vi "Teleop.vi"(10 "Match Info":T1={"Autonomous Elapsed Seconds"=0.0, "TeleOp Elapsed Seconds"=0.0, "Disabled Elapsed Seconds"=0.0, "Visited Autonomous"=FALSE, "Visited TeleOp"=FALSE, "Visited Disabled"=FALSE, "Autonomous Settings"={"Autonomous Style"=enum."Independent", "VI Refnum"=refnum}}, 11 "Call Context":T2) -> ()   [LabVIEW 2014]
doc: "This VI is called for each TeleOp packet received from the DS where the robot is not disabled. It is often used to read from the joysticks and update I/O or to update setpoints for timed control loops. It should complete and return within 20 milliseconds or it may miss DS packets."
uses:
  <vilib>/Rock Robotics/WPI/DriverStation/WPI_DriverStationDerivedRobotMode.ctl
  <vilib>/Rock Robotics/WPI/DriverStation/WPI_DriverStationMatch Info.ctl
  <vilib>/Rock Robotics/Network Tables/SD Read Boolean.vi
  <vilib>/Rock Robotics/Network Tables/SD Read Number.vi
  <vilib>/Rock Robotics/WPI/RobotDrive/WPI_RobotDriveGetSetRefNum.vi
  <vilib>/Rock Robotics/WPI/Joystick/WPI_JoystickGetSetRefNum.vi
  <vilib>/Rock Robotics/Network Tables/SD Write Boolean Array.vi
  <vilib>/Rock Robotics/Network Tables/SD Write Numeric Array.vi
  <vilib>/Rock Robotics/WPI/RobotDrive/WPI_RobotDriveArcadeDrive_Standard(NoSaturation).vi
  Robot Global Data.vi
  <vilib>/Rock Robotics/WPI/Solenoid/WPI_SolenoidValue.ctl
  <vilib>/addons/control/pid/NI_PID_pid.lvlib
  <vilib>/Rock Robotics/WPI/Solenoid/WPI_SolenoidSetEnum.vi
  <vilib>/addons/control/pid/pid.llb/PID (DBL).vi
panel:
  out "EncoderDistance":dbl
  out "GyroAngle":dbl
  out "ArmVoltage":dbl
  out "Sample Slider 0":dbl(slide) scale=0.0..5.0
  out "Sample Boolean 1":bool
  out "Sample Boolean 0":bool
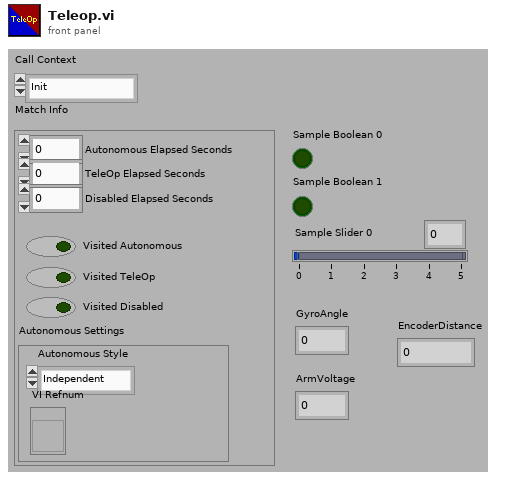
[diagram p1: front panel]
types:
  T1 = typedef "WPI_DriverStationMatch Info.ctl" = cluster{"Autonomous Elapsed Seconds":dbl, "TeleOp Elapsed Seconds":dbl, "Disabled Elapsed Seconds":dbl, "Visited Autonomous":bool, "Visited TeleOp":bool, "Visited Disabled":bool, "Autonomous Settings":cluster{"Autonomous Style":enum16{"Iterative", "Independent"}, "VI Refnum":refnum<vi>}}
  T2 = typedef "WPI_DriverStationDerivedRobotMode.ctl" = enum16{"Init", "Execute", "Stop"}
  T3 = typedef "WPI_JoystickDevRef.ctl" = cluster{"Device":T4}
  T4 = typedef "WPI_JoystickDeviceEnum.ctl" = enum16{"USB 0", "USB 1", "USB 2", "USB 3", "USB 4", "USB 5"}
  T5 = typedef "WPI_SolenoidValue.ctl" = enum16{"Off", "On", "Forward", "Reverse"}
  T6 = typedef "WPI_SolenoidDevRef.ctl" = cluster{"DevStatus":errorcluster, "Pneumatics Control Module":u8, "Forward Solenoid Channel":T7, "Reverse Solenoid Channel":T7}
  T7 = typedef "WPI_SolenoidChannel.ctl" = enum8{"Solenoid 0", "Solenoid 1", "Solenoid 2", "Solenoid 3", "Solenoid 4", "Solenoid 5", "Solenoid 6", "Solenoid 7", "Invalid"}
  T8 = cluster{"proportional gain (Kc)":dbl, "integral time (Ti, min)":dbl, "derivative time (Td, min)":dbl}
  T9 = typedef "WPI_AnalogChannelDevRef.ctl" = cluster{"DevStatus":errorcluster, "Controller":T10, "Analog Channel":T11}
  T10 = typedef "FPGA_TypedefAnalogModule.ctl" = enum16{"Controller 1"}
  T11 = typedef "FPGA_AIChannel.ctl" = enum8{"AI 0", "AI 1", "AI 2", "AI 3", "AI MXP 0", "AI MXP 1", "AI MXP 2", "AI MXP 3", "Invalid"}
  T12 = typedef "WPI_MotorControlDeviceRef.ctl" = cluster{"DeviceStatus":errorcluster, "Type":T13, "PWM":cluster{"Controller":T14, "PWM Channel":T15, "DeadBand":T16}, "CAN":cluster{"Device Number":u8, "Control Mode":T17, "Semaphore":T18, "Max Vout":dbl, "TalonSRX Control Mode":T19}, "Invert":bool, "TransformRef":T20, "InvTransformRef":T20}
  T13 = typedef "WPI_MotorControlType.ctl" = enum16{"PWM", "CAN", "CANTalonSRX"}
  T14 = typedef "FPGA_TypedefDigitalModule.ctl" = enum16{"Controller 1"}
  T15 = typedef "FPGA_DIOPWMChannel.ctl" = enum8{"PWM 0", "PWM 1", "PWM 2", "PWM 3", "PWM 4", "PWM 5", "PWM 6", "PWM 7", "PWM 8", "PWM 9", "PWM MXP 0", "PWM MXP 1", "PWM MXP 2", "PWM MXP 3", "PWM MXP 4", "PWM MXP 5", "PWM MXP 6", "PWM MXP 7", "PWM MXP 8", "PWM MXP 9", "Invalid"}
  T16 = typedef "WPI_PWMDeadband.ctl" = cluster{"Name":string, "maxPositivePwm":i32, "minPositivePwm":i32, "centerPwm":i32, "maxNegativePwm":i32, "minNegativePwm":i32, "angularRange":u16}
  T17 = typedef "WPI_CANJaguar_ControlMode.ctl" = enum8{"Percent VBus", "Current", "Speed", "Position", "Voltage"}
  T18 = typedef "Semaphore RefNum" = refnum<k1>
  T19 = typedef "WPI_CANTalonSRX_APIControlMode.ctl" = enum8{"Percent VBus", "Speed", "Position", "Slave", "Unchanged / Invalid"}
  T20 = typedef "WPI_PWMTransform_ConPane.ctl" = refnum<vi>
  T21 = typedef "WPI_RobotDriveDevRef.ctl" = cluster{"DevStatus":errorcluster, "Motors[]":T12[], "Square Inputs":bool, "Max Output":dbl}
  T22 = typedef "WPI_GyroDevRef.ctl" = cluster{"DevStatus":errorcluster, "Analog Module":T10, "Analog Channel":T11, "Offset":dbl, "Gain (VoltsPerDegree/Second)":dbl}
  T23 = typedef "WPI_EncoderDevRef.ctl" = cluster{"DevStatus":errorcluster, "EncoderIndex":T24, "CounterIndex":T25, "DistancePerCount":dbl, "Decoding Type":T26}
  T24 = typedef "FPGA_EncoderIdx.ctl" = enum8{"Enc 0", "Enc 1", "Enc 2", "Enc 3", "Enc 4", "Enc 5", "Enc 6", "Enc 7", "Invalid"}
  T25 = typedef "FPGA_CounterCtrSystemIndex.ctl" = enum8{"Ctr 0", "Ctr 1", "Ctr 2", "Ctr 3", "Ctr 4", "Ctr 5", "Ctr 6", "Ctr 7", "Invalid"}
  T26 = typedef "WPI_EncoderType.ctl" = enum16{"1x", "2x", "4x"}
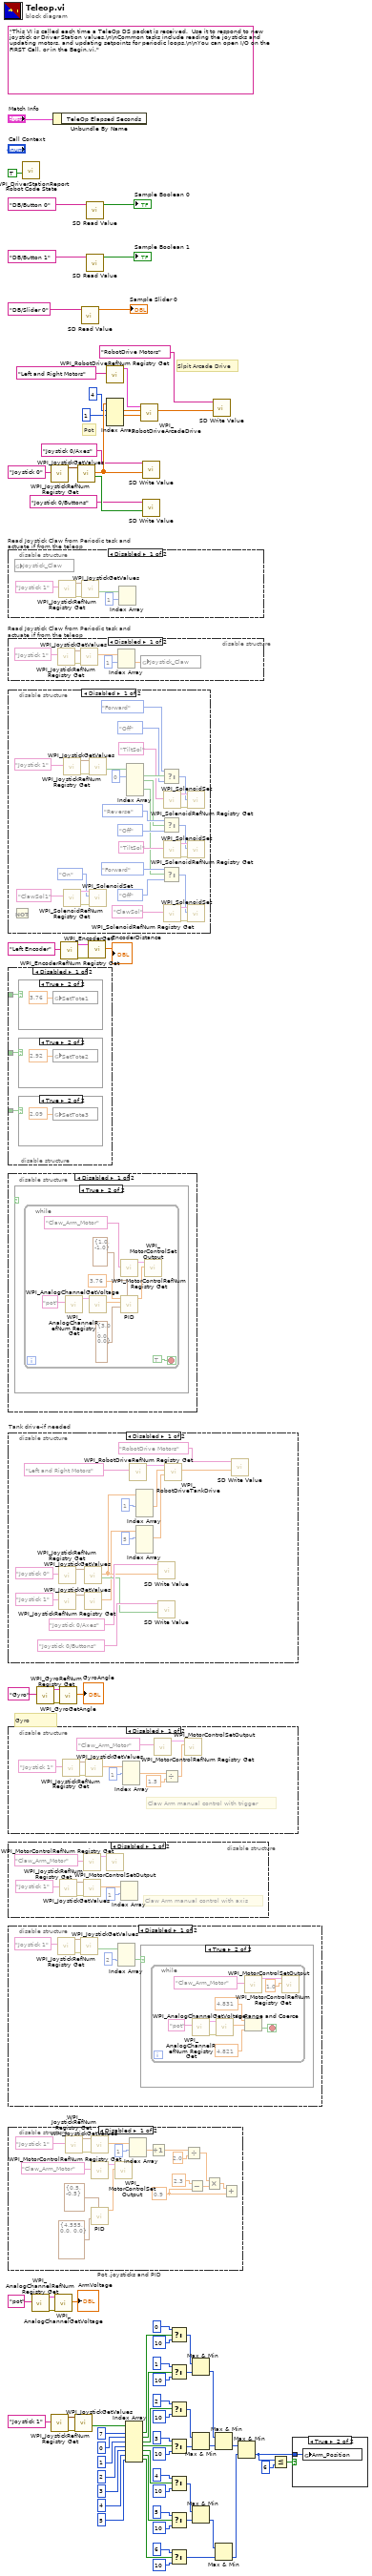
[diagram p0: block diagram]
diagram:
  (unwired) "This VI is called each time a TeleOp DS packet is received.  Use it to respond to new joystick or Driver Station values.\n\nCommon tasks include reading the joysticks and updating motors, and updating setpoints for periodic loops.\n\nYou can open I/O on the FIRST Call, or in the Begin.vi."
  # "Gyro"
  # "Pot"
  # "Slpit Arcade Drive"
  n1 = disable-structure "Read Joystick Claw from Periodic task and actuate if from the teleop" shown="Disabled" {
    frame Disabled {
      n2 = global read "Robot Global Data.vi" "Joystick_Claw"() -> ()  [unwired: 1 in]
      n3 = call <vilib>:"WPI_JoystickRefNum Registry Get.vi"("refnum name"="Joystick 1") -> ("error out"=w85:errorcluster, "JoystickDevRef"=w84:T3)  [unwired: 1 in, 8 out]
      n4 = call <vilib>:"WPI_JoystickGetValues.vi"("error in (no error)"=w85, "JoystickDevRef"=w84) -> ("Buttons"=w82:bool[])  [unwired: 5 in, 4 out]
      n5 = Index Array(array=w82, index #1=1 ("index")) -> ()  [unwired: 1 in, 2 out]
    }
    frame Enabled {
    }
  }
  n6 = disable-structure "Read Joystick Claw from Periodic task and actuate if from the teleop" shown="Disabled" {
    frame Disabled {
      n7 = call <vilib>:"WPI_JoystickRefNum Registry Get.vi"("refnum name"="Joystick 1") -> ("error out"=w90:errorcluster, "JoystickDevRef"=w89:T3)  [unwired: 1 in, 8 out]
      n8 = call <vilib>:"WPI_JoystickGetValues.vi"("error in (no error)"=w90, "JoystickDevRef"=w89) -> ("Axes"=w91:dbl[])  [unwired: 5 in, 4 out]
      n9 = Index Array(array=w91, index #1=1 ("index")) -> (element #1=w87:dbl)  [unwired: 1 in, 1 out]
      n10 = global write "Robot Global Data.vi" "Joystick_Claw"(w87) -> ()
    }
    frame Enabled {
    }
  }
  n11 = disable-structure shown="Disabled" {
    frame Disabled {
      n12 = Not() -> ()  [unwired: 1 in, 1 out]
      n13 = call <vilib>:"WPI_JoystickRefNum Registry Get.vi"("refnum name"="Joystick 1") -> ("error out"=w120:errorcluster, "JoystickDevRef"=w119:T3)  [unwired: 9 in]
      n14 = call <vilib>:"WPI_SolenoidRefNum Registry Get.vi"("refnum name"="ClawSol1") -> ("error out"=w101:errorcluster, "SolenoidDevRef"=w102:T6)  [unwired: 9 in]
      n15 = call <vilib>:"WPI_JoystickGetValues.vi"("error in (no error)"=w120, "JoystickDevRef"=w119) -> ("Buttons"=w112:bool[])  [unwired: 5 in, 4 out]
      n16 = call-poly <vilib>:"WPI_SolenoidSet.vi"("error in (no error)"=w101, "Value"=WPI_SolenoidValue."On", "SolenoidDevRef"=w102) -> ()  [unwired: 7 in, 2 out]
      n17 = Index Array(array=w112, index #1=0 ("index")) -> (element #1=w117:bool, element #2=w104:bool, element #4=w94:bool)  [unwired: 4 in, 2 out]
      n18 = Select(t=WPI_SolenoidValue."Forward", s=w117, f=WPI_SolenoidValue."Off" ("Value")) -> (s? t:f=w115:T5)
      n19 = Select(t=WPI_SolenoidValue."Reverse", s=w104, f=WPI_SolenoidValue."Off" ("Value")) -> (s? t:f=w107:T5)
      n20 = Select(t=WPI_SolenoidValue."Forward", s=w94, f=WPI_SolenoidValue."Off" ("Value")) -> (s? t:f=w97:T5)
      n21 = call <vilib>:"WPI_SolenoidRefNum Registry Get.vi"("refnum name"="TiltSol") -> ("error out"=w122:errorcluster, "SolenoidDevRef"=w121:T6)  [unwired: 9 in]
      n22 = call <vilib>:"WPI_SolenoidRefNum Registry Get.vi"("refnum name"="TiltSol") -> ("error out"=w108:errorcluster, "SolenoidDevRef"=w109:T6)  [unwired: 9 in]
      n23 = call <vilib>:"WPI_SolenoidRefNum Registry Get.vi"("refnum name"="ClawSol") -> ("error out"=w100:errorcluster, "SolenoidDevRef"=w99:T6)  [unwired: 9 in]
      n24 = call-poly <vilib>:"WPI_SolenoidSet.vi"("error in (no error)"=w122, "Value"=w115, "SolenoidDevRef"=w121) -> ()  [unwired: 7 in, 2 out]
      n25 = call-poly <vilib>:"WPI_SolenoidSet.vi"("error in (no error)"=w108, "Value"=w107, "SolenoidDevRef"=w109) -> ()  [unwired: 7 in, 2 out]
      n26 = call-poly <vilib>:"WPI_SolenoidSet.vi"("error in (no error)"=w100, "Value"=w97, "SolenoidDevRef"=w99) -> ()  [unwired: 7 in, 2 out]
    }
    frame Enabled {
    }
  }
  n27 = disable-structure shown="Disabled" {
    disable-tunnel: _ -> [w125 _]
    disable-tunnel: _ -> [w124 _]
    disable-tunnel: _ -> [w123 _]
    frame Disabled {
      n28 = case shown="True" w125 {
        frame False {
        }
        frame True {
          n29 = global write "Robot Global Data.vi" "SetTote1"(3.76 ("SetTote1")) -> ()
        }
      }
      n30 = case shown="True" w124 {
        frame False {
        }
        frame True {
          n31 = global write "Robot Global Data.vi" "SetTote2"(2.92 ("SetTote2")) -> ()
        }
      }
      n32 = case shown="True" w123 {
        frame False {
        }
        frame True {
          n33 = global write "Robot Global Data.vi" "SetTote3"(2.09 ("SetTote3")) -> ()
        }
      }
    }
    frame Enabled {
    }
  }
  n34 = disable-structure shown="Disabled" {
    frame Disabled {
      n35 = case shown="True" {
        selector: _ -> [_ _]
        frame False {
        }
        frame True {
          n36 = while {
            stop <- TRUE stop-if-true
            n37 = call <vilib>:"WPI_AnalogChannelRefNum Registry Get.vi"("refnum name"="pot") -> ("AIDeviceRef"=w132:T9)  [unwired: 9 in, 1 out]
            n38 = call <vilib>:"WPI_AnalogChannelGetVoltage.vi"("AIDeviceRef"=w132) -> ("Voltage"=w138:dbl)  [unwired: 1 in, 9 out]
            n39 = call <vilib>:"WPI_MotorControlRefNum Registry Get.vi"("refnum name"="Claw_Arm_Motor") -> ("MotorControlDevRef"=w135:T12)  [unwired: 1 in, 9 out]
            n40 = call-poly <vilib>:"PID.vi"("output range"=cluster{"output high":dbl, "output low":dbl} {"output high"=1.0, "output low"=-1.0}, "PID gains"=T8 {"proportional gain (Kc)"=3.0, "integral time (Ti, min)"=0.0, "derivative time (Td, min)"=0.0}, "process variable"=w138, "setpoint"=3.76 ("SetTote1")) -> ("output"=w130:dbl)  [unwired: 2 in, 5 out]
            n41 = call <vilib>:"WPI_MotorControlSetOutput.vi"("Output"=w130, "MotorControlDevRef"=w135) -> ()  [unwired: 2 in, 8 out]
          }
        }
      }
    }
    frame Enabled {
    }
  }
  n42 = disable-structure "Tank drive-if needed" shown="Disabled" {
    frame Disabled {
      n43 = call <vilib>:"WPI_JoystickRefNum Registry Get.vi"("refnum name"="Joystick 0") -> ("JoystickDevRef"=w153:T3)  [unwired: 1 in, 9 out]
      n44 = call <vilib>:"WPI_JoystickRefNum Registry Get.vi"("refnum name"="Joystick 1") -> ("JoystickDevRef"=w143:T3)  [unwired: 1 in, 9 out]
      n45 = call <vilib>:"WPI_JoystickGetValues.vi"("JoystickDevRef"=w143) -> ("Axes"=w144:dbl[])  [unwired: 6 in, 4 out]
      n46 = call <vilib>:"WPI_JoystickGetValues.vi"("JoystickDevRef"=w153) -> ("Buttons"=w148:bool[], "Axes"=w150:dbl[])  [unwired: 6 in, 3 out]
      n47 = call <vilib>:"WPI_RobotDriveRefNum Registry Get.vi"("refnum name"="Left and Right Motors") -> ("RobotDriveDevRef"=w147:T21)  [unwired: 1 in, 9 out]
      n48 = Index Array(array=w150, index #2=1 ("index")) -> (element #2=w145:dbl)  [unwired: 3 in, 3 out]
      n49 = Index Array(array=w144, index #1=5 ("index")) -> (element #1=w140:dbl)  [unwired: 3 in, 3 out]
      n50 = call-poly <vilib>:"SD Write Value.vi"("Numeric Array"=w150, "Name"="Joystick 0/Axes") -> ()  [unwired: 8 in, 2 out]
      n51 = call-poly <vilib>:"SD Write Value.vi"("Boolean Array"=w148, "Name"="Joystick 0/Buttons") -> ()  [unwired: 8 in, 2 out]
      n52 = call <vilib>:"WPI_RobotDriveTankDrive.vi"("Right axis value"=w140, "Left axis value"=w145, "RobotDriveDevRef"=w147) -> ("Motor Values"=w139:dbl[])  [unwired: 6 in, 2 out]
      n53 = call-poly <vilib>:"SD Write Value.vi"("Numeric Array"=w139, "Name"="RobotDrive Motors") -> ()  [unwired: 8 in, 2 out]
    }
    frame Enabled {
    }
  }
  n54 = disable-structure shown="Disabled" {
    frame Disabled {
      # "Claw Arm manual control with trigger"
      n55 = call <vilib>:"WPI_JoystickRefNum Registry Get.vi"("refnum name"="Joystick 1") -> ("error out"=w163:errorcluster, "JoystickDevRef"=w164:T3)  [unwired: 1 in, 8 out]
      n56 = call <vilib>:"WPI_JoystickGetValues.vi"("error in (no error)"=w163, "JoystickDevRef"=w164) -> ("Axes"=w160:dbl[])  [unwired: 5 in, 4 out]
      n57 = Index Array(array=w160, index #1=1 ("index")) -> (element #1=w158:dbl)  [unwired: 2 in, 2 out]
      n58 = call <vilib>:"WPI_MotorControlRefNum Registry Get.vi"("refnum name"="Claw_Arm_Motor") -> ("MotorControlDevRef"=w161:T12)  [unwired: 1 in, 9 out]
      n59 = Divide(x=w158, y=1.5) -> (x/y=w156:dbl)
      n60 = call <vilib>:"WPI_MotorControlSetOutput.vi"("Output"=w156, "MotorControlDevRef"=w161) -> ()  [unwired: 2 in, 8 out]
    }
    frame Enabled {
    }
  }
  n61 = disable-structure shown="Disabled" {
    frame Disabled {
      # "Claw Arm manual control with axis"
      n62 = call <vilib>:"WPI_JoystickRefNum Registry Get.vi"("refnum name"="Joystick 1") -> ("error out"=w168:errorcluster, "JoystickDevRef"=w167:T3)  [unwired: 1 in, 8 out]
      n63 = call <vilib>:"WPI_MotorControlRefNum Registry Get.vi"("refnum name"="Claw_Arm_Motor") -> ("MotorControlDevRef"=w170:T12)  [unwired: 1 in, 9 out]
      n64 = call <vilib>:"WPI_JoystickGetValues.vi"("error in (no error)"=w168, "JoystickDevRef"=w167) -> ("Axes"=w171:dbl[])  [unwired: 5 in, 4 out]
      n65 = call <vilib>:"WPI_MotorControlSetOutput.vi"("MotorControlDevRef"=w170) -> ()  [unwired: 3 in, 8 out]
      n66 = Index Array(array=w171, index #1=1 ("index")) -> ()  [unwired: 1 in, 2 out]
    }
    frame Enabled {
    }
  }
  n67 = disable-structure shown="Disabled" {
    frame Disabled {
      n68 = call <vilib>:"WPI_JoystickRefNum Registry Get.vi"("refnum name"="Joystick 1") -> ("error out"=w176:errorcluster, "JoystickDevRef"=w177:T3)  [unwired: 1 in, 8 out]
      n69 = call <vilib>:"WPI_JoystickGetValues.vi"("error in (no error)"=w176, "JoystickDevRef"=w177) -> ("Buttons"=w175:bool[])  [unwired: 5 in, 4 out]
      n70 = Index Array(array=w175, index #2=2 ("index")) -> (element #2=w174:bool)  [unwired: 2 in, 2 out]
      n71 = case shown="True" w174 {
        frame False {
        }
        frame True {
          n72 = while {
            stop <- w179 stop-if-true
            n73 = call <vilib>:"WPI_AnalogChannelRefNum Registry Get.vi"("refnum name"="pot") -> ("error out"=w185:errorcluster, "AIDeviceRef"=w184:T9)  [unwired: 9 in]
            n74 = call <vilib>:"WPI_AnalogChannelGetVoltage.vi"("error in (no error)"=w185, "AIDeviceRef"=w184) -> ("Voltage"=w180:dbl)  [unwired: 7 in, 2 out]
            n75 = call <vilib>:"WPI_MotorControlRefNum Registry Get.vi"("refnum name"="Claw_Arm_Motor") -> ("MotorControlDevRef"=w187:T12)  [unwired: 1 in, 9 out]
            n76 = In Range and Coerce(upper limit=4.831 ("lower limit"), x=w180, lower limit=4.821 ("upper limit")) -> (In Range?=w179:bool)  [unwired: 1 out]
            n77 = call <vilib>:"WPI_MotorControlSetOutput.vi"("Output"=1.0, "MotorControlDevRef"=w187) -> ()  [unwired: 2 in, 8 out]
          }
        }
      }
    }
    frame Enabled {
    }
  }
  n78 = disable-structure "Pot ,joysticks and PID" shown="Disabled" {
    frame Disabled {
      w194 = 0.9 ("y")
      n79 = call <vilib>:"WPI_JoystickRefNum Registry Get.vi"("refnum name"="Joystick 1") -> ("error out"=w204:errorcluster, "JoystickDevRef"=w203:T3)  [unwired: 1 in, 8 out]
      n80 = call <vilib>:"WPI_JoystickGetValues.vi"("error in (no error)"=w204, "JoystickDevRef"=w203) -> ("Axes"=w205:dbl[])  [unwired: 5 in, 4 out]
      n81 = call <vilib>:"WPI_MotorControlRefNum Registry Get.vi"("refnum name"="Claw_Arm_Motor") -> ("MotorControlDevRef"=w193:T12)  [unwired: 1 in, 9 out]
      n82 = call-poly <vilib>:"PID.vi"("output range"=cluster{"output high":dbl, "output low":dbl} {"output high"=0.5, "output low"=-0.5}, "PID gains"=T8 {"proportional gain (Kc)"=4.555, "integral time (Ti, min)"=0.0, "derivative time (Td, min)"=0.0}) -> ("output"=w189:dbl)  [unwired: 8 in, 1 out]
      n83 = call <vilib>:"WPI_MotorControlSetOutput.vi"("Output"=w189, "MotorControlDevRef"=w193) -> ()  [unwired: 2 in, 8 out]
      n84 = Index Array(array=w205, index #1=1 ("index")) -> (element #1=w201:dbl)  [unwired: 1 in, 1 out]
      n85 = Increment(x=w201) -> (x+1=w200:dbl)
      n86 = Divide(x=w200, y=2.0) -> (x/y=w198:dbl)
      n87 = Subtract(x=2.3, y=w194) -> (x-y=w197:dbl)
      n88 = Multiply(x=w198, y=w197) -> (x*y=w195:dbl)
      n89 = Add(x=w195, y=w194) -> ()  [unwired: 1 out]
    }
    frame Enabled {
    }
  }
  n90 = call <vilib>:"WPI_DriverStationReport Robot Code State.vi"("TeleOp"=TRUE ("Autonomous")) -> ()  [unwired: 10 in, 1 out]
  n91 = call <vilib>:"WPI_AnalogChannelRefNum Registry Get.vi"("refnum name"="pot") -> ("error out"=w54:errorcluster, "AIDeviceRef"=w55:T9)  [unwired: 9 in]
  n92 = call <vilib>:"WPI_GyroRefNum Registry Get.vi"("refnum name"="Gyro") -> ("error out"=w60:errorcluster, "GyroDevRef"=w59:T22)  [unwired: 9 in]
  n93 = call <vilib>:"WPI_JoystickRefNum Registry Get.vi"("refnum name"="Joystick 0") -> ("JoystickDevRef"=w67:T3)  [unwired: 1 in, 9 out]
  n94 = call <vilib>:"WPI_JoystickRefNum Registry Get.vi"("refnum name"="Joystick 1") -> ("error out"=w49:errorcluster, "JoystickDevRef"=w4:T3)  [unwired: 1 in, 8 out]
  n95 = Unbundle By Name("Match Info") -> ()  [unwired: 1 out]
  n96 = call <vilib>:"WPI_AnalogChannelGetVoltage.vi"("error in (no error)"=w54, "AIDeviceRef"=w55) -> ("Voltage"=→"ArmVoltage":dbl)  [unwired: 7 in, 2 out]
  n97 = call <vilib>:"WPI_GyroGetAngle.vi"("error in (no error)"=w60, "GyroDevRef"=w59) -> ("Angle"=→"GyroAngle":dbl)  [unwired: 6 in, 3 out]
  n98 = call <vilib>:"WPI_EncoderRefNum Registry Get.vi"("refnum name"="Left Encoder") -> ("error out"=w3:errorcluster, "EncoderDevRef"=w2:T23)  [unwired: 9 in]
  n99 = call <vilib>:"WPI_JoystickGetValues.vi"("error in (no error)"=w49, "JoystickDevRef"=w4) -> ("Buttons"=w47:bool[])  [unwired: 5 in, 4 out]
  n100 = call <vilib>:"WPI_JoystickGetValues.vi"("JoystickDevRef"=w67) -> ("Buttons"=w72:bool[], "Axes"=w70:dbl[])  [unwired: 6 in, 3 out]
  n101 = call-poly <vilib>:"SD Read Value.vi"("Name"="DB/Slider 0" ("refnum name")) -> ("Numeric"=→"Sample Slider 0":dbl)  [unwired: 8 in, 2 out]
  n102 = call-poly <vilib>:"SD Read Value.vi"("Name"="DB/Button 0" ("refnum name")) -> ("Boolean"=→"Sample Boolean 0":bool)  [unwired: 8 in, 2 out]
  n103 = call-poly <vilib>:"SD Read Value.vi"("Name"="DB/Button 1" ("refnum name")) -> ("Boolean"=→"Sample Boolean 1":bool)  [unwired: 8 in, 2 out]
  n104 = call <vilib>:"WPI_EncoderGet.vi"("error in (no error)"=w3, "EncoderDevRef"=w2) -> ("Distance"=→"EncoderDistance":dbl)  [unwired: 4 in, 5 out]
  n105 = call <vilib>:"WPI_RobotDriveRefNum Registry Get.vi"("refnum name"="Left and Right Motors") -> ("RobotDriveDevRef"=w73:T21)  [unwired: 1 in, 9 out]
  n106 = Index Array(array=w70, index #1=4 ("index"), index #2=1 ("index")) -> (element #1=w64:dbl, element #2=w63:dbl)  [unwired: 2 in, 2 out]
  n107 = Index Array(array=w47, index #1=7 ("index"), index #2=0 ("index"), index #3=1 ("index"), index #4=2 ("index"), index #5=3 ("index"), index #6=4 ("index"), index #7=5 ("index")) -> (element #1=w44:bool, element #2=w36:bool, element #3=w35:bool, element #4=w34:bool, element #5=w33:bool, element #6=w32:bool, element #7=w31:bool)
  n108 = call-poly <vilib>:"WPI_RobotDriveArcadeDrive.vi"("Y axis value"=w63, "X axis value"=w64, "RobotDriveDevRef"=w73) -> ("Motor Values"=w74:dbl[])  [unwired: 6 in, 2 out]
  n109 = call-poly <vilib>:"SD Write Value.vi"("Numeric Array"=w70, "Name"="Joystick 0/Axes") -> ()  [unwired: 8 in, 2 out]
  n110 = call-poly <vilib>:"SD Write Value.vi"("Boolean Array"=w72, "Name"="Joystick 0/Buttons") -> ()  [unwired: 8 in, 2 out]
  n111 = Select(t=0, s=w44, f=10) -> (s? t:f=w43:i32)
  n112 = Select(t=1, s=w36, f=10) -> (s? t:f=w25:i32)
  n113 = Select(t=2, s=w35, f=10) -> (s? t:f=w19:i32)
  n114 = Select(t=3, s=w34, f=10) -> (s? t:f=w20:i32)
  n115 = Select(t=4, s=w33, f=10) -> (s? t:f=w22:i32)
  n116 = Select(t=5, s=w32, f=10) -> (s? t:f=w23:i32)
  n117 = Select(t=6, s=w31, f=10) -> (s? t:f=w24:i32)
  n118 = Max & Min(x=w43, y=w25) -> (min(x,y)=w18:i32)  [unwired: 1 out]
  n119 = Max & Min(x=w19, y=w20) -> (min(x,y)=w17:i32)  [unwired: 1 out]
  n120 = Max & Min(x=w22, y=w23) -> (min(x,y)=w21:i32)  [unwired: 1 out]
  n121 = call-poly <vilib>:"SD Write Value.vi"("Numeric Array"=w74, "Name"="RobotDrive Motors") -> ()  [unwired: 8 in, 2 out]
  n122 = Max & Min(x=w18, y=w17) -> (min(x,y)=w16:i32)  [unwired: 1 out]
  n123 = Max & Min(x=w21, y=w24) -> (min(x,y)=w15:i32)  [unwired: 1 out]
  n124 = Max & Min(x=w16, y=w15) -> (min(x,y)=w7:i32)  [unwired: 1 out]
  n125 = Less Or Equal?(x=w7, y=6) -> (x <= y?=w5:bool)
  n126 = case shown="True" w5 {
    tunnel: w7 -> [_ w207]
    frame False {
    }
    frame True {
      n127 = global write "Robot Global Data.vi" "Arm_Position"(w207) -> ()
    }
  }
